vi "Reset Communication.vi"(8 "error in":errorcluster, 10 "Node-ID":u8, 11 "Network Management in":refnum<class "Network Management.lvclass">) -> (0 "error out":errorcluster, 3 "Network Management out":refnum<class "Network Management.lvclass">)   [LabVIEW 2020, in "CANopen.lvlib" / "Network Management.lvlib" / "Network Management.lvclass"]
uses:
  Network Management.lvclass
  Network Management.lvclass/Network Management.ctl
  CANopen Message/CANopen Message.lvclass
  Typedefs/Function Code.ctl
  CANopen.lvlib
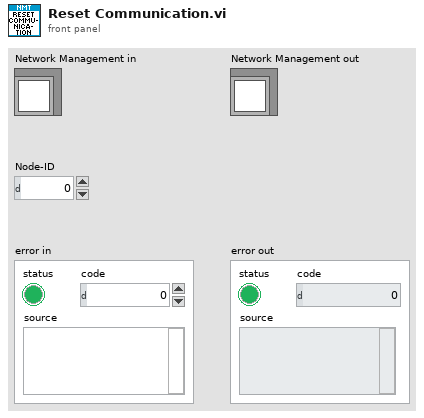
[diagram p1: front panel]
types:
  T1 = typedef "CANopen.lvlib/Function Code.ctl" = u8
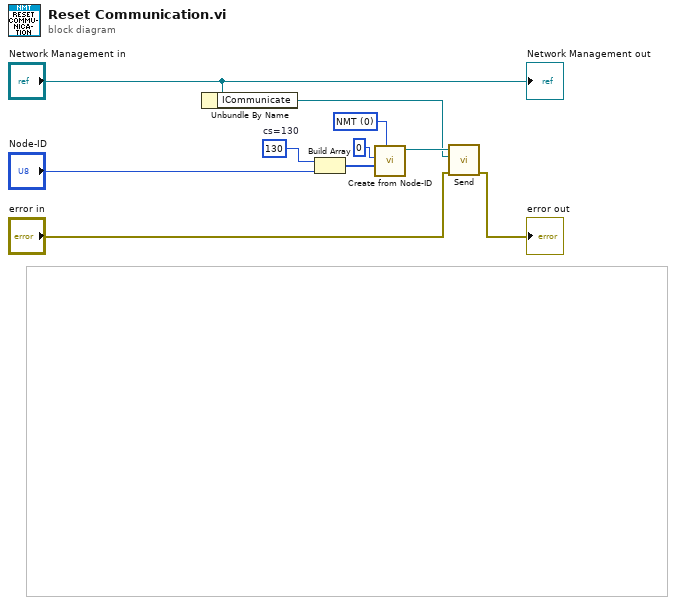
[diagram p0: block diagram]
diagram:
  w8 = u8 130  # cs=130
  w9 = T1 0 items=["NMT"=0, "EMCY/SYNC"=1, "TIME"=2, "PDO1 (tx)"=3, "PDO1 (rx)"=4, "PDO2 (tx)"=5, "PDO2 (rx)"=6, "PDO3 (tx)"=7, "PDO3 (rx)"=8, "PDO4 (tx)"=9, "PDO4 (rx)"=10, "SDO (tx)"=11, "SDO (rx)"=12, "NMT error control"=14] ("Function Code")
  n1 = Unbundle By Name("Network Management in") -> ("ICommunicate"=w3:refnum<class "ICommunicate.lvclass">)
  n2 = Build Array(w8, "Node-ID") -> (w6:u8[])
  n3 = call "Create from Node-ID.vi"("Function Code"=w9, "Data"=w6, "Node-ID"=u8 0) -> ("CANopen Message"=w4:refnum<class "CANopen Message.lvclass">)  [unwired: 8 in]
  n4 = call "Send.vi"("error in"="error in", "ICommunicate"=w3, "CANopen Message in"=w4) -> ("error out"=→"error out":errorcluster)  [unwired: 7 in, 1 out]
  "Network Management out" <- "Network Management in"
